vi "GUI_channelTable.vi"(5 "ref channels table":refnum<vi>, 7 "ref spectrum channel type":refnum<vi>, 8 "error in (no error)":errorcluster, 10 "dataType":T1, 11 "Thorlabs_OSA_64 in":refnum<class "OSA.lvclass">) -> (0 "error out":errorcluster, 3 "Thorlabs_OSA_64 out":refnum<class "OSA.lvclass">)   [LabVIEW 2010, in "OSA.lvclass"]
uses:
  OSA.lvclass
  typeDef/acq_dataType.ctl
  OSA20X_misc.lvlib
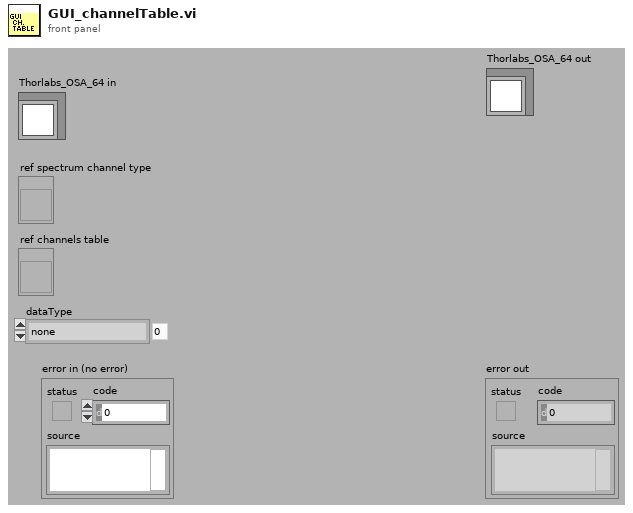
[diagram p1: front panel]
types:
  T1 = typedef "OSA.lvclass/acq_dataType.ctl" = enum16{"none", "interferogram", "spectrum"}
  T2 = enum8{"Enabled", "Disabled", "Disabled and Grayed Out"}
  T3 = typedef "OSA20X_misc.lvlib/channel_propertiesGen.ctl" = cluster{"waveMin (cm-1)":sgl, "waveMax (cm-1)":sgl, "gain levels nr":u16, "offset max":u16, "detector sort":T4, "adc #bits":u16, "temp Variable":bool, "wavemtrOn":bool, "offset":i32, "offset max":u16, "damperAvailable":bool, "damperActive":bool, "damperAuto":bool, "gainOffset auto":bool}
  T4 = typedef "OSA20X_misc.lvlib/detector_sort.ctl" = enum16{"unknown", "Silicon", "Silicon PIN", "Silicon MPPC", "InGaAs", "InGaAs ext low", "InGaAs ext high", "InAs", "InAsSb", "InSb", "MCT", "other", "other2", "other3"}
  T5 = typedef "OSA20X_misc.lvlib/channelType_spectrum.ctl" = enum16{"SINGLE CHANNEL", "STICHED"}
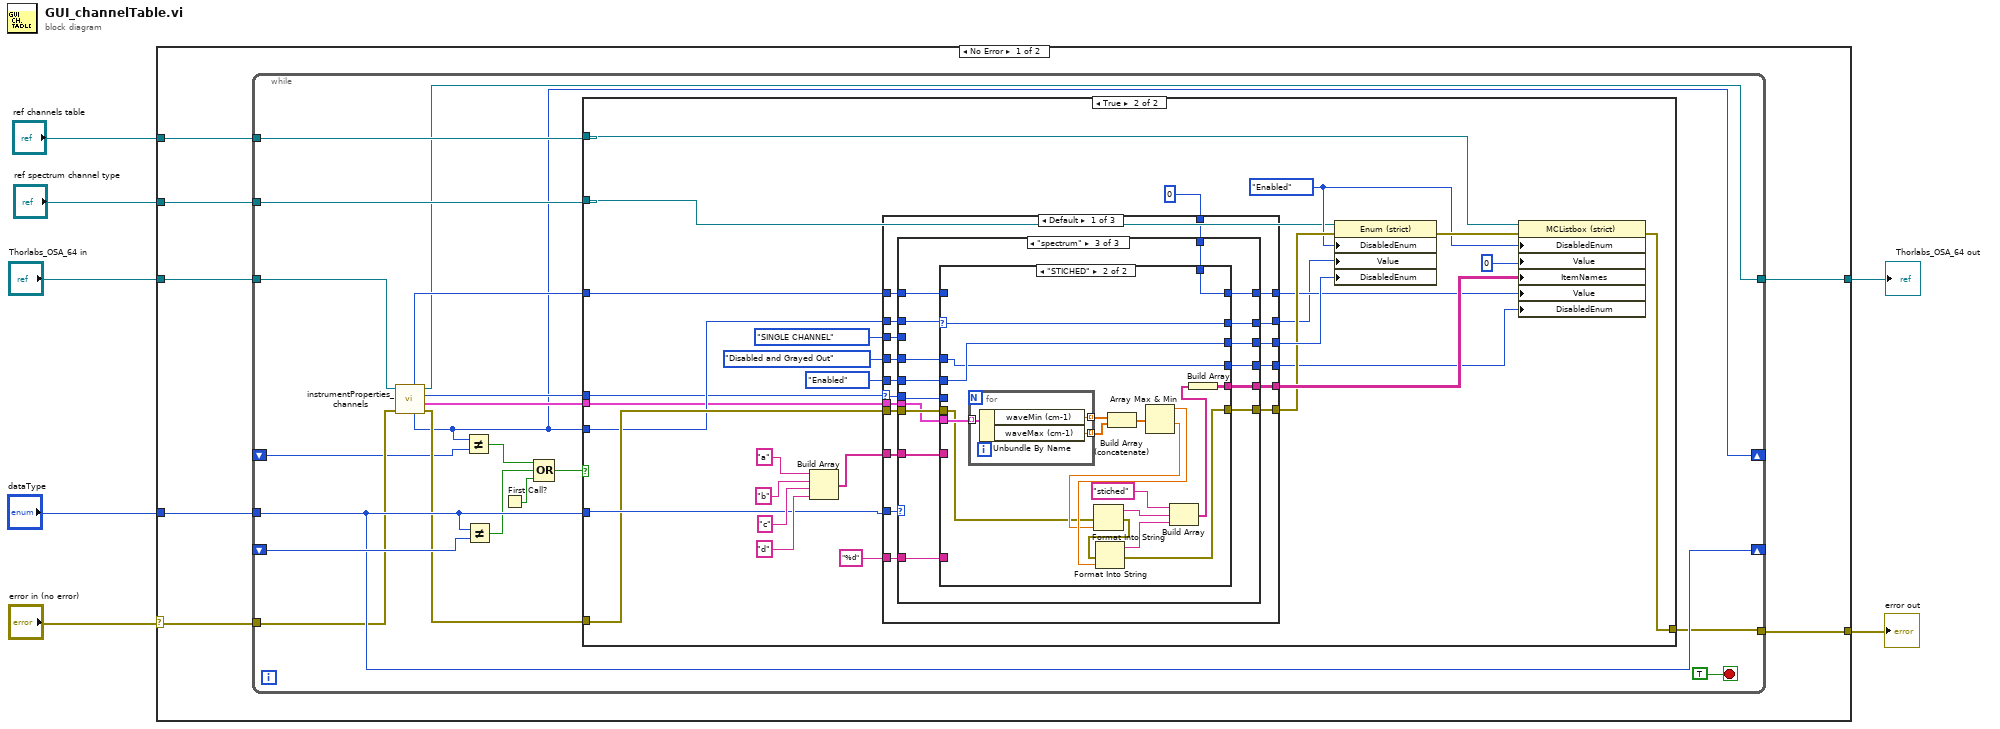
[diagram p0: block diagram]
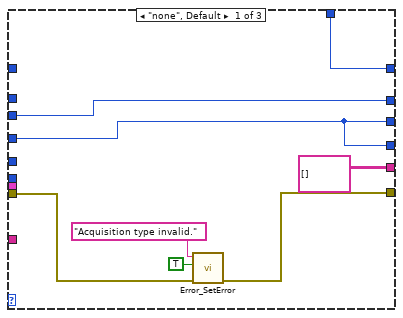
[diagram p3: hidden frame]
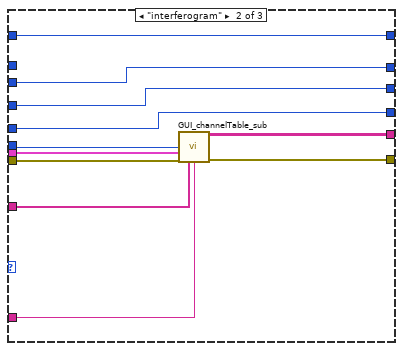
[diagram p4: hidden frame]
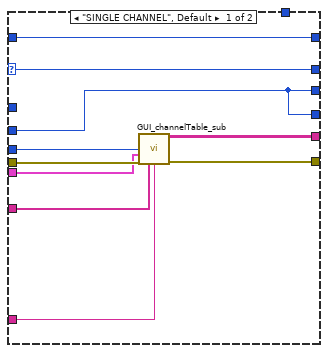
[diagram p5: hidden frame]
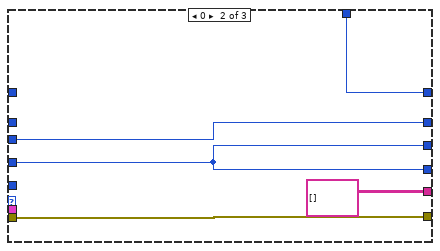
[diagram p6: hidden frame]
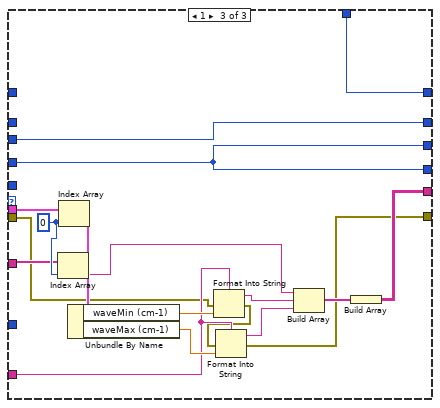
[diagram p7: hidden frame]
diagram:
  n1 = case shown="No Error" "error in (no error)" {
    selector: "error in (no error)" -> [w13 w171]
    tunnel: [w9 w171] -> w6
    tunnel: [w12 w170] -> w4
    tunnel: "Thorlabs_OSA_64 in" -> [w14 w170]
    tunnel: "ref spectrum channel type" -> [w8 _]
    tunnel: "ref channels table" -> [w10 _]
    tunnel: "dataType" -> [w11 _]
    frame No Error {
      n2 = while {
        tunnel: w14 -> [w27]
        tunnel: w13 -> [w26]
        tunnel: [w22] -> w12
        tunnel: w11 -> [w31]
        tunnel: w10 -> [w29]
        tunnel: [w28] -> w9
        tunnel: w8 -> [w30]
        shift-right: [w31] -> _
        shift-left: _ -> [w33]
        shift-right: [w15] -> _
        shift-left: _ -> [w16]
        stop <- TRUE stop-if-true
        n3 = call-dynamic "instrumentProperties_channels.vi"("error in (no error)"=w26, "Thorlabs_OSA_64 in"=w27) -> ("error out"=w25:errorcluster, "channel properties"=w23:T3[], "channels nr"=w21:i32, "Thorlabs_OSA_64 out"=w22:refnum<class "OSA.lvclass">, "spectrum channel type"=w15:T5, "channel DUT (index)"=w24:i32)  [unwired: 4 in]
        n4 = Not Equal?(x=w15, y=w16) -> (x != y?=w20:bool)
        n5 = Not Equal?(x=w31, y=w33) -> (x != y?=w19:bool)
        n6 = First Call?() -> (First Call?: T/F=w18:bool)
        n7 = Compound Arithmetic op=OR(w20, w19, w18) -> (w17:bool)
        n8 = case shown="True" w17 {
          tunnel: w25 -> [w34 w38]
          tunnel: w29 -> [_ w62]
          tunnel: [w34 w44] -> w28
          tunnel: w30 -> [_ w41]
          tunnel: w31 -> [_ w40]
          tunnel: w24 -> [_ w39]
          tunnel: w15 -> [_ w37]
          tunnel: w23 -> [_ w36]
          tunnel: w21 -> [_ w35]
          frame False {
          }
          frame True {
            w42 = T2."Enabled" ("Disabled")
            n9 = Build Array("a" ("element"), "b" ("element"), "c" ("element"), "d" ("element")) -> (w54:string[])
            n10 = case shown="Default" w35 {
              selector: w35 -> [w79 _ _]
              tunnel: w36 -> [w80 _ w169]
              tunnel: [w70 w150 w168] -> w43
              tunnel: enum16{"SINGLE CHANNEL", "STICHED"}."SINGLE CHANNEL" ("Value") -> [w71 w150 w168]
              tunnel: [w72 w148 w153] -> w59
              tunnel: T2."Disabled and Grayed Out" ("Disabled") -> [w73 w148 w153]
              tunnel: w38 -> [w76 w149 w158]
              tunnel: [w75 string[][] [] w156] -> w50
              tunnel: w54 -> [w77 _ w161]
              tunnel: T2."Enabled" ("Disabled") -> [w67 _ _]
              tunnel: "%d" ("format string") -> [w78 _ w159]
              tunnel: w40 -> [w74 _ _]
              tunnel: [w69 w149 w154] -> w48
              tunnel: w37 -> [w68 _ _]
              tunnel: [w63 w148 w153] -> w47
              tunnel: [w66 w147 w152] -> w46
              tunnel: 0 ("Value") -> [w64 w147 w152]
              tunnel: w39 -> [w65 _ _]
              frame Default {
                n11 = case shown="\"spectrum\"" w74 {
                  tunnel: w80 -> [_ w94 w109]
                  tunnel: w79 -> [_ w93 w110]
                  tunnel: w78 -> [_ w96 w112]
                  tunnel: w77 -> [_ w95 w111]
                  tunnel: w76 -> [w86 w98 w114]
                  tunnel: [string[][] [] ("table strings") w92 w108] -> w75
                  tunnel: w73 -> [w81 w99 w100]
                  tunnel: [w81 w99 w106] -> w72
                  tunnel: w71 -> [w83 w91 _]
                  tunnel: [w83 w91 w107] -> w70
                  tunnel: [w85 w97 w113] -> w69
                  tunnel: w68 -> [_ _ w115]
                  tunnel: w67 -> [_ w89 w105]
                  tunnel: [w82 w90 w104] -> w66
                  tunnel: w65 -> [_ w90 w103]
                  tunnel: w64 -> [w82 _ w102]
                  tunnel: [w81 w89 w101] -> w63
                  frame "none", Default {
                    n12 = call "Error_SetError.vi"("error in"=w86, "status (true)"=TRUE, "source(\"\")"="Acquisition type invalid." ("source(\"\")")) -> ("error out"=w85:errorcluster)  [unwired: 4 in]
                  }
                  frame "interferogram" {
                    n13 = call "GUI_channelTable_sub.vi"("channels nr"=w93, "channel properties"=w94, "error in"=w98, "col0 strings"=w95, "format string"=w96) -> ("table strings"=w92:string[][], "error out"=w97:errorcluster)  [unwired: 9 in]
                  }
                  frame "spectrum" {
                    n14 = case shown="\"STICHED\"" w115 {
                      selector: w115 -> [w118 w129]
                      tunnel: w114 -> [w125 w134]
                      tunnel: [w124 w133] -> w113
                      tunnel: w112 -> [w123 _]
                      tunnel: w111 -> [w122 _]
                      tunnel: w110 -> [w121 _]
                      tunnel: w109 -> [w120 w140]
                      tunnel: [w119 w130] -> w108
                      tunnel: [w118 w129] -> w107
                      tunnel: [w116 w128] -> w106
                      tunnel: w105 -> [w116 w128]
                      tunnel: [w117 w127] -> w104
                      tunnel: w103 -> [w117 _]
                      tunnel: w102 -> [_ w127]
                      tunnel: [w116 w126] -> w101
                      tunnel: w100 -> [_ w126]
                      frame "SINGLE CHANNEL", Default {
                        n15 = call "GUI_channelTable_sub.vi"("channels nr"=w121, "channel properties"=w120, "error in"=w125, "col0 strings"=w122, "format string"=w123) -> ("table strings"=w119:string[][], "error out"=w124:errorcluster)  [unwired: 9 in]
                      }
                      frame "STICHED" {
                        n16 = for {
                          tunnel: w140 -> [w146] mode=indexing
                          tunnel: [w145] -> w138 mode=indexing
                          tunnel: [w144] -> w139 mode=indexing
                          n17 = Unbundle By Name(w146) -> ("waveMin (cm-1)"=w145:sgl, "waveMax (cm-1)"=w144:sgl)
                        }
                        n18 = Build Array (concatenate)(w138, w139) -> (w137:sgl[])
                        n19 = Array Max & Min(array=w137) -> (max value=w136:sgl, min value=w135:sgl)  [unwired: 2 out]
                        n20 = Format Into String(error in=w134, w135) -> (resulting string=w143:string, error out=w141:errorcluster)  [unwired: 2 in]
                        n21 = Format Into String(error in=w141, w136) -> (resulting string=w142:string, error out=w133:errorcluster)  [unwired: 2 in]
                        n22 = Build Array("stiched" ("element"), w143, w142) -> (w131:string[])
                        n23 = Build Array(w131) -> (w130:string[][])
                      }
                    }
                  }
                }
              }
              frame 0 {
              }
              frame 1 {
                w162 = 0 ("index")
                n24 = Index Array(array=w161, index=w162) -> (element=w160:string)
                n25 = Index Array(array=w169, index=w162) -> (element=w167:T3)
                n26 = Unbundle By Name(w167) -> ("waveMin (cm-1)"=w166:sgl, "waveMax (cm-1)"=w165:sgl)
                n27 = Format Into String(format string=w159, error in=w158, w166) -> (resulting string=w164:string, error out=w157:errorcluster)  [unwired: 1 in]
                n28 = Format Into String(format string=w159, error in=w157, w165) -> (resulting string=w163:string, error out=w154:errorcluster)  [unwired: 1 in]
                n29 = Build Array(w160, w164, w163) -> (w155:string[])
                n30 = Build Array(w155) -> (w156:string[][])
              }
            }
            n31 = property class="Enum (strict)"(reference=w41, error in=w48, "DisabledEnum"=w42, "Value"=w43, "DisabledEnum"=w59) -> (error out=w51:errorcluster)  [unwired: 1 out]
            n32 = property class="MCListbox (strict)"(reference=w62, error in=w51, "DisabledEnum"=w42, "Value"=0, "ItemNames"=w50, "Value"=w46, "DisabledEnum"=w47) -> (error out=w44:errorcluster)  [unwired: 1 out]
          }
        }
      }
    }
    frame Error {
    }
  }
  "error out" <- w6
  "Thorlabs_OSA_64 out" <- w4
